vi "MM9.get library version.vi"() -> (0 "nameAndVersion":string)   [LabVIEW 2014, in "MM9.lvlib"]
doc: "obtain name and version of a library as a string"
uses:
  MM9.lvlib
  CSlibraries/UtilityLib/UtilityLib.lvlib
  LEBITLib/LEBITLib.lvlib
  LEBITDefs9/LEBITDefs9.lvlib
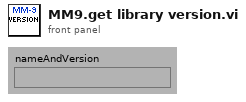
[diagram p1: front panel]
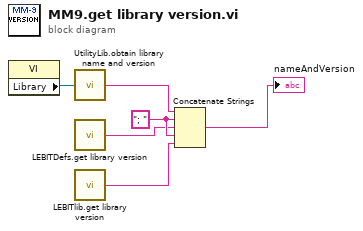
[diagram p0: block diagram]
diagram:
  w3 = "; " ("string")
  n1 = property class="VI"() -> ("Library"=w6:refnum<vi>)  [unwired: 2 in, 2 out]
  n2 = call "UtilityLib.obtain library name and version.vi"("Library"=w6) -> ("nameAndVersion"=w5:string)
  n3 = call "LEBITDefs.get library version.vi"() -> ("nameAndVersion"=w2:string)  [unwired: 1 in]
  n4 = call "LEBITlib.get library version.vi"() -> ("nameAndVersion"=w1:string)  [unwired: 1 in]
  n5 = Concatenate Strings(w5, w3, w2, w3, w1) -> (→"nameAndVersion":string)
